vi "Too Many VISA Sessions.vi"(11 "Threshold":i32=256) -> (3 "Number of Open VISA Sessions":i32)   [LabVIEW 2021]
doc: "VI to detect when number of VISA sessions is growing out of control. Defaults to error with 256 VISA sessions and pops up MODAL dialog box.\nScott Hannahs <sth@magnet.fsu.edu>\nMarch 2023"
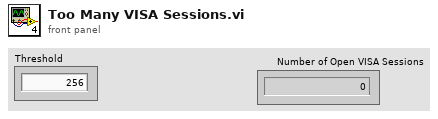
[diagram p1: front panel]
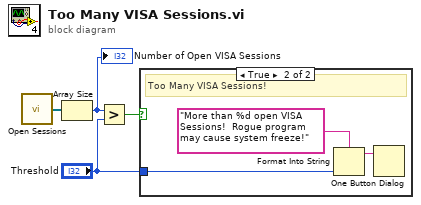
[diagram p0: block diagram]
diagram:
  n1 = call <vilib>:"Open Sessions.vi"() -> ("Array of Refnums"=w4:refnum<visa-resource-name>[])  [unwired: 2 in]
  n2 = Array Size(array=w4) -> (size(s)=w2:i32)
  "Number of Open VISA Sessions" <- w2
  n3 = Greater?(x=w2, y="Threshold") -> (0:w3:bool)
  n4 = case shown="True" w3 {
    tunnel: "Threshold" -> [_ w6]
    frame False {
    }
    frame True {
      # "Too Many VISA Sessions!"
      n5 = Format Into String(format string="More than %d open VISA Sessions!  Rogue program may cause system freeze!" ("message"), w6) -> (resulting string=w7:string)  [unwired: 2 in, 1 out]
      n6 = One Button Dialog(message=w7) -> ()  [unwired: 1 in, 1 out]
    }
  }
